vi "goToV0.vi"(10 "RobotModelAllInformation in":T1, 11 "Robot in":refnum<class "Robot.lvclass">) -> (2 "RobotModelAllInformation out":T1, 3 "Robot out":refnum<class "Robot.lvclass">)   [LabVIEW 2023, in "Game.lvclass"]
uses:
  Game.lvclass
  Controls/RobotModelAllInformation.ctl
  Controls/RobotModelTestCrashCase.ctl
  VelocityPlanningTest/Controls/robotModelArray.ctl
  Controls/RobotModel.ctl
  Robot_class/Robot.lvclass
  Robot_class/Robot.lvclass/Robot.ctl
  Robot_class/Read est_v_tang.vi
  Robot_class/Write v_tang.vi
  Robot_class/Write v_norm.vi
  Robot_class/Write v_ang.vi
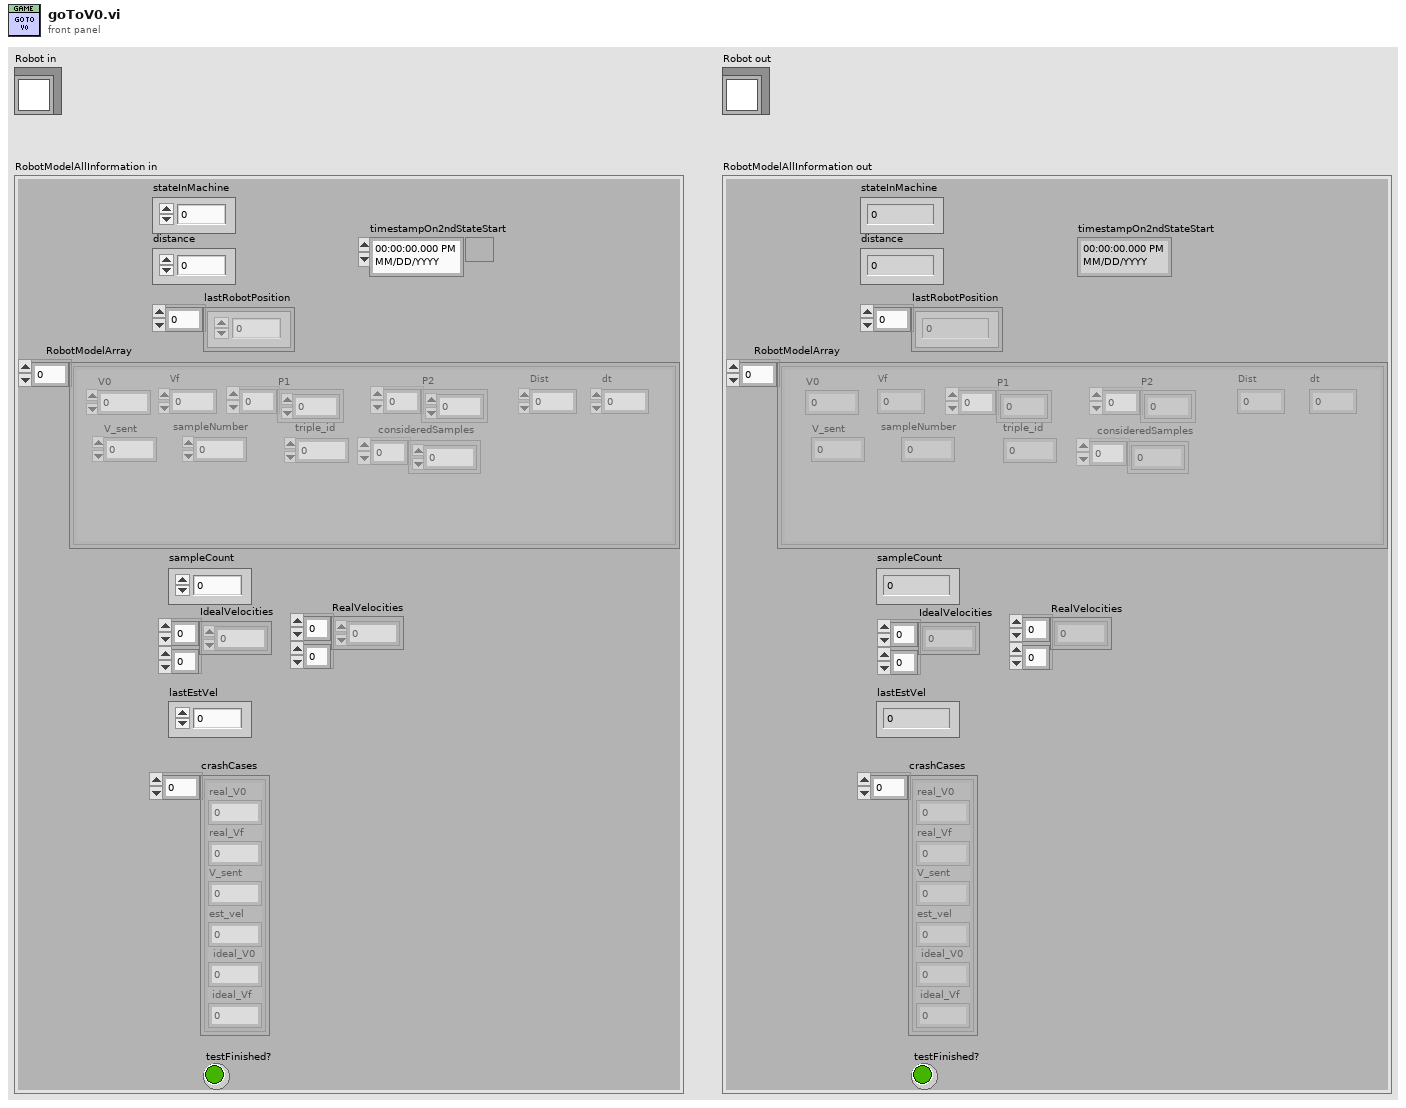
[diagram p1: front panel]
types:
  T1 = typedef "RobotModelAllInformation.ctl" = cluster{"distance":dbl, "lastRobotPosition":dbl[], "timestampOn2ndStateStart":timestamp, "sampleCount":i32, "stateInMachine":i32, "crashCases":T2[], "lastEstVel":dbl, "IdealVelocities":dbl[][], "RealVelocities":dbl[][], "testFinished?":bool, "RobotModelArray":T3}
  T2 = typedef "RobotModelTestCrashCase.ctl" = cluster{"real_V0":dbl, "real_Vf":dbl, "V_sent":dbl, "est_vel":dbl, "ideal_V0":dbl, "ideal_Vf":dbl}
  T3 = typedef "robotModelArray.ctl" = T4[]
  T4 = typedef "RobotModel.ctl" = cluster{"V0":dbl, "Vf":dbl, "Dist":dbl, "dt":dbl, "P1":dbl[], "P2":dbl[], "V_sent":dbl, "sampleNumber":i32, "triple_id":i32, "consideredSamples":dbl[]}
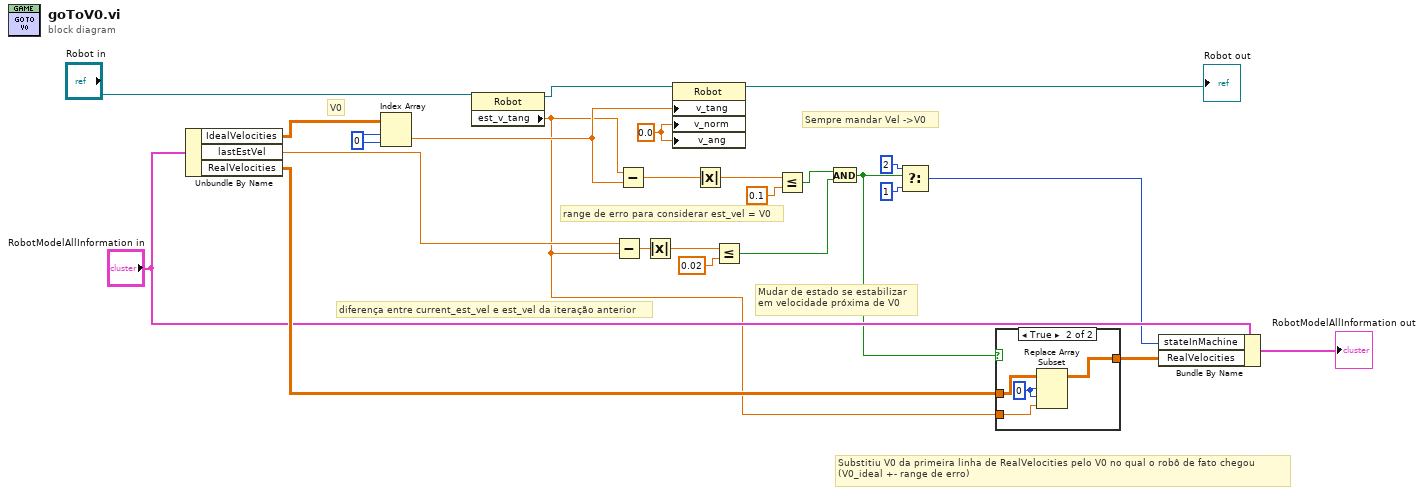
[diagram p0: block diagram]
diagram:
  w23 = 0 ("index (row)")
  w1 = 0.0 ("v_norm")
  # "Substitiu V0 da primeira linha de RealVelocities pelo V0 no qual o robô de fato chegou\n(V0_ideal +- range de erro)"
  # "diferença entre current_est_vel e est_vel da iteração anterior"
  # "range de erro para considerar est_vel = V0"
  # "V0"
  # "Mudar de estado se estabilizar\nem velocidade próxima de V0"
  # "Sempre mandar Vel ->V0"
  n1 = Unbundle By Name("RobotModelAllInformation in") -> ("IdealVelocities"=w22:dbl[][], "lastEstVel"=w21:dbl, "RealVelocities"=w25:dbl[][])
  n2 = Index Array(array=w22, index (row)=w23, index (col)=w23) -> (element=w24:dbl)
  n3 = property class="Robot"(reference="Robot in") -> (reference out=w2:refnum<class "Robot.lvclass">, "est_v_tang"=w14:dbl)  [unwired: 1 in, 1 out]
  n4 = Subtract(x=w21, y=w14) -> (x-y=w9:dbl)
  n5 = Subtract(x=w14, y=w24) -> (x-y=w10:dbl)
  n6 = Absolute Value(x=w9) -> (abs(x)=w3:dbl)
  n7 = property class="Robot"(reference=w2, "v_tang"=w24, "v_norm"=w1, "v_ang"=w1) -> (reference out=→"Robot out":refnum<class "Robot.lvclass">)  [unwired: 1 in, 1 out]
  n8 = Absolute Value(x=w10) -> (abs(x)=w12:dbl)
  n9 = Less Or Equal?(x=w3, y=0.02) -> (x <= y?=w16:bool)
  n10 = Less Or Equal?(x=w12, y=0.1) -> (x <= y?=w15:bool)
  n11 = And(x=w15, y=w16) -> (x .and. y?=w13:bool)
  n12 = Select(t=2, s=w13, f=1) -> (s? t:f=w18:i32)
  n13 = case shown="True" w13 {
    tunnel: w25 -> [w26 w30]
    tunnel: [w26 w28] -> w17
    tunnel: w14 -> [_ w29]
    frame False {
    }
    frame True {
      w27 = 0 ("index")
      n14 = Replace Array Subset(array=w30, new element=w29, index (row)=w27, index (col)=w27) -> (w28:dbl[][])
    }
  }
  n15 = Bundle By Name(cluster="RobotModelAllInformation in", "stateInMachine"=w18, "RealVelocities"=w17) -> (→"RobotModelAllInformation out":T1)
